vi "Edge Detection.vi"() -> ()   [LabVIEW 2014]
doc: "This example shows how to use the Edge Tool in NI Vision. The Edge Tool finds edges (or sharp transitions in the pixels values) along a given line or ROI profile. The Edge Tool is a precursor function to many of the gauging and inspection tasks. For example, the location of the edges found along a line profile across an object can interpreted as the boundaries of the object whose dimensions have to be measured for a gauging application or the presence of a crack in the surface of an object for an inspection application."
uses:
  <vilib>/vision/NI_Vision_Development_Module.lvlib
panel:
  out "Number of Edges Detected":i32
  in  "Process":u16(ring)=2 items=["Get First Edge", "Get First + Last Edge", "Get All Edges", "Get Best Edge"]
  in  "Edge Options":T1={"Edge Polarity"=0, "Kernel Size"=3, "Width"=5, "Minimum Edge Strength"=10.0, "Interpolation Type"=1, "Data Processing Method"=0} {"Data Processing Method" items=["Average", "Median"]; "Interpolation Type" items=["Zero Order"=0, "Bilinear"=1, "Bilinear Fixed"=4]; "Minimum Edge Strength" min=0.0 max=255.0 format="%.2g"; "Width" min=1 step=2; "Kernel Size" min=3 step=2; "Edge Polarity" items=["All Edges", "Rising Edges", "Falling Edges"]}
  out "Gradient Information":dbl[](graph)
  out "Image":T2(plugin-control)
  out "Line Profile":cluster{"x0":sgl, "dx":sgl, "Pixels Line":sgl[]}(graph)
  in  "Stop":bool
  # "Overview: Demonstrates how to use the IMAQ Edge Tool function to find edges along a Region of Interest (ROI).\nRequirements: Vision Development Software.\nInstructions:\n1. Run the VI.\n2. Draw a ROI in the image or change the Process or Edge Options to see the edges detected along the ROI."
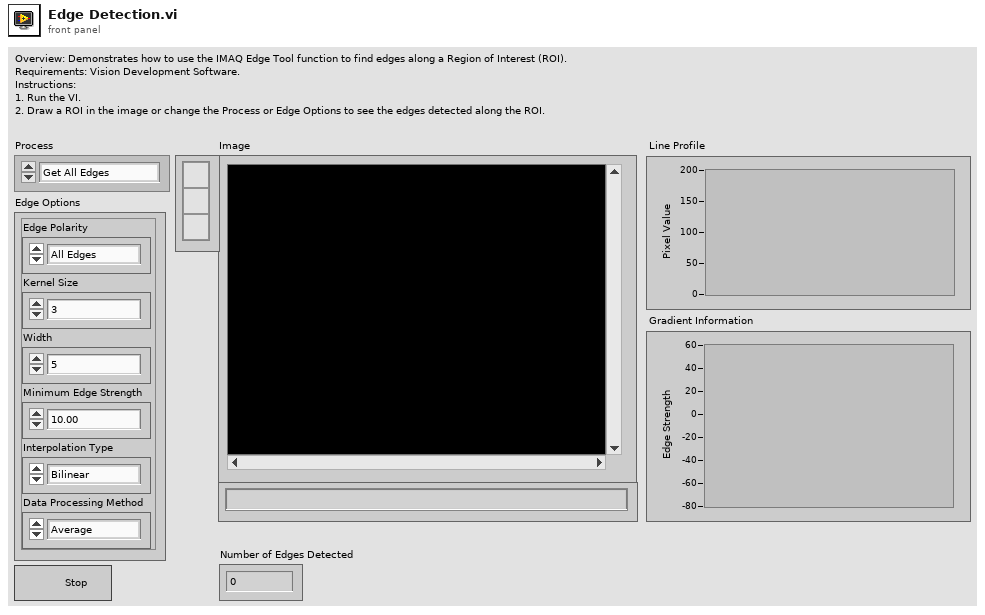
[diagram p1: front panel]
types:
  T1 = cluster{"Edge Polarity":u16, "Kernel Size":u32, "Width":u32, "Minimum Edge Strength":dbl, "Interpolation Type":u16, "Data Processing Method":u16}
  T2 = typedef "IMAQ Image.ctl" = refnum<image>
  T3 = typedef "IMAQ Line" = cluster{"Start X":i32, "Start Y":i32, "End X":i32, "End Y":i32}
  T4 = typedef "ROI Descriptor" = cluster{"Global Rectangle":i32[], "Contours":cluster{"ID":enum32{"External", "Internal"}, "Type":u32, "Coordinates":i32[]}[]}
  T5 = cluster{"Global Rectangle":i32[], "Contours":cluster{"Contour Type":u32, "ROI Type":u32, "Points":i32[]}[]}
  T6 = typedef "Edge New.ctl" = cluster{"Location (Pixel)":cluster{"X":sgl, "Y":sgl}, "Location (Real-World)":cluster{"X":sgl, "Y":sgl}, "Distance (Pixel)":dbl, "Distance (Real-World)":dbl, "Strength":dbl, "Noise":dbl, "Rising?":bool}
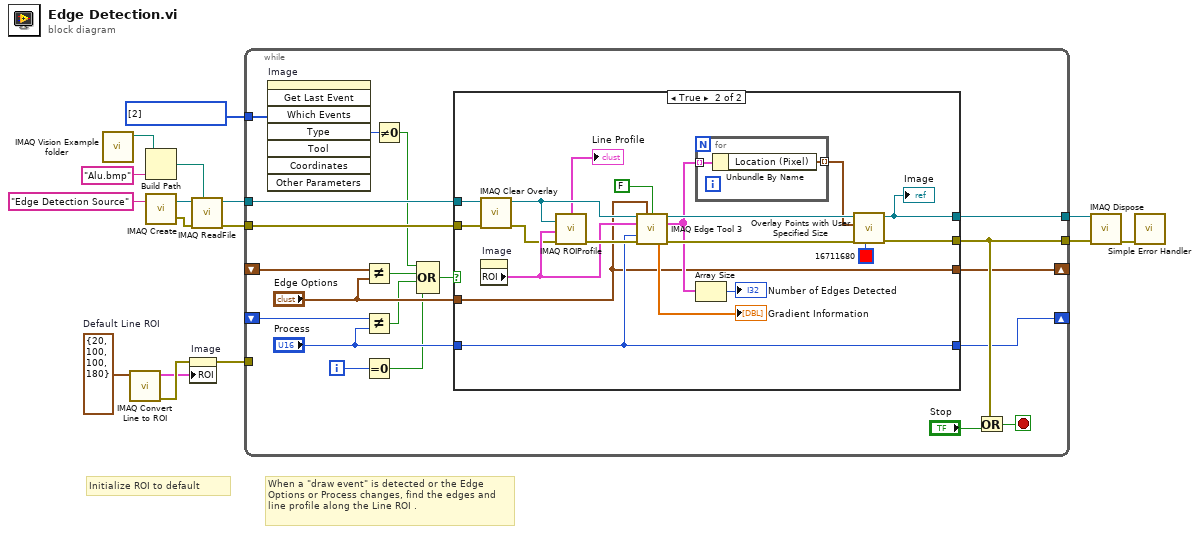
[diagram p0: block diagram]
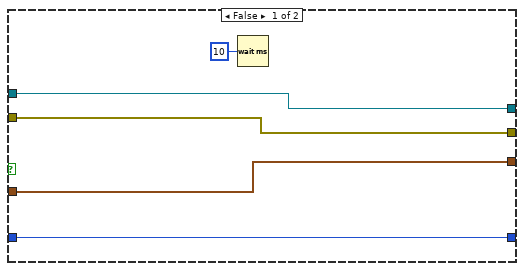
[diagram p2: hidden frame]
diagram:
  w4 = T3 {"Start X"=20, "Start Y"=100, "End X"=100, "End Y"=180}  # Default Line ROI
  w5 = i32[] [2] items=["No  event", "Click event", "Draw event", "Move event", "Size event", "Scroll event", "Activate event", "Close event", "Double click event"] ("Events list (all)")
  # "Initialize ROI to default"
  # "When a \"draw event\" is detected or the Edge Options or Process changes, find the edges and line profile along the Line ROI ."
  n1 = call "IMAQ Vision Example folder.vi"() -> ("Example Image Path"=w15:path)  [unwired: 11 in]
  n2 = call "IMAQ Convert Line to ROI"("Line"=w4) -> ("error out"=w3:errorcluster, "ROI Descriptor"=w2:T4)  [unwired: 8 in]
  n3 = Build Path(base path=w15, name or relative path="Alu.bmp") -> (appended path=w11:path)
  n4 = call "IMAQ Create"("Image Name"="Edge Detection Source") -> ("New Image"=w13:T2, "error out"=w12:errorcluster)  [unwired: 4 in]
  n5 = property on="Image" class="ImageControl"(error in=w3, "ROI"=w2) -> (error out=w1:errorcluster)  [unwired: 1 in, 1 out]
  n6 = call "IMAQ ReadFile"("File Path"=w11, "error in (no error)"=w12, "Image"=w13) -> ("error out"=w6:errorcluster, "Image Out"=w7:T2)  [unwired: 4 in, 3 out]
  n7 = while {
    tunnel: w7 -> [w35]
    tunnel: w6 -> [w36]
    tunnel: [w31] -> w10
    tunnel: [w32] -> w9
    tunnel: w5 -> [w30]
    shift-right: [w17] -> _
    shift-left: _ -> [w27]
    shift-right: [w18] -> _
    shift-left: _ -> [w25]
    tunnel: w1 -> [_]
    i -> [w28]
    stop <- w33 stop-if-true
    n8 = invoke on="Image" class="ImageControl" method="Get Last Event"("Which Events"=w30) -> ("Type"=w29:i32)  [unwired: 7 in, 7 out]
    n9 = Not Equal?(x=w27, y="Edge Options") -> (x != y?=w23:bool)
    n10 = Not Equal?(x=w25, y="Process") -> (x != y?=w22:bool)
    n11 = Equal To 0?(x=w28) -> (x = 0?=w21:bool)
    n12 = Not Equal To 0?(x=w29) -> (x != 0?=w20:bool)
    n13 = Compound Arithmetic op=OR(w20, w23, w22, w21) -> (w19:bool)
    n14 = case shown="True" w19 {
      tunnel: w36 -> [w40 w50]
      tunnel: w35 -> [w41 w49]
      tunnel: [w41 w52] -> w32
      tunnel: [w40 w56] -> w31
      tunnel: "Edge Options" -> [w38 w43]
      tunnel: "Process" -> [w37 w45]
      tunnel: [w37 w45] -> w18
      tunnel: [w38 w43] -> w17
      frame False {
        n15 = Wait (ms)(milliseconds to wait=u32 10) -> ()  [unwired: 1 out]
      }
      frame True {
        n16 = call "IMAQ Clear Overlay"("error in (no error)"=w50, "Image"=w49) -> ("error out"=w47:errorcluster, "Image Out"=w48:T2)  [unwired: 8 in]
        n17 = property on="Image" class="ImageControl"() -> ("ROI"=w51:T5)  [unwired: 2 in, 2 out]
        n18 = call "IMAQ ROIProfile"("error in (no error)"=w47, "ROI Descriptor"=w51, "Image"=w48) -> ("error out"=w58:errorcluster, "ROI Graph"=→"Line Profile":cluster{"x0":sgl, "dx":sgl, "Pixels Line":sgl[]})  [unwired: 1 in, 3 out]
        n19 = call "IMAQ Edge Tool 3"("Image"=w48, "Edge Options"=w43, "Optimized Mode"=FALSE, "ROI Descriptor"=w51, "Process"=w45, "error in (no error)"=w58) -> ("Image (duplicate)"=w55:T2, "Edge Information"=w54:T6[], "Gradient Values"=→"Gradient Information":dbl[], "error out"=w57:errorcluster)  [unwired: 5 in, 1 out]
        n20 = for {
          tunnel: w54 -> [w62] mode=indexing
          tunnel: [w61] -> w42 mode=indexing
          n21 = Unbundle By Name(w62) -> ("Location (Pixel)"=w61:cluster{"X":sgl, "Y":sgl})
        }
        n22 = Array Size(array=w54) -> (size(s)=→"Number of Edges Detected":i32)
        n23 = call "Overlay Points with User Specified Size.vi"("Color"=u32 16711680, "error in"=w57, "Points"=w42, "Image In"=w55) -> ("error out"=w56:errorcluster, "Image Out"=w52:T2)  [unwired: 6 in]
        "Image" <- w52
      }
    }
    n24 = Or(x=w31, y="Stop") -> (x .or. y?=w33:bool)
  }
  n25 = call "IMAQ Dispose"("Image"=w9, "error in (no error)"=w10) -> ("error out"=w8:errorcluster)  [unwired: 4 in]
  n26 = call <vilib>:"Simple Error Handler.vi"("error in (no error)"=w8) -> ()  [unwired: 4 in, 5 out]
